vi "JSON FASES GEN.vi"(5 "time":u32, 7 "Tension":dbl, 8 "error in":errorcluster, 9 "Fase":u32, 10 "Corriente":dbl, 11 "Potencia":dbl) -> (0 "error out":errorcluster, 3 "JSON Object out":refnum<class "JSON Object.lvclass">)   [LabVIEW 2015]
uses:
  <vilib>/addons/JSON API/Get Polymorphic/JSON GetSet.lvlib
  <vilib>/addons/JSON API/JSON Scalar/Set SGL.vi
  <vilib>/addons/JSON API/JSON Scalar/JSON Scalar.lvclass
  <vilib>/addons/JSON API/JSON Object/Set Object Item by name.vi
  <vilib>/addons/JSON API/JSON Object/JSON Object.lvclass
  <vilib>/addons/JSON API/JSON Scalar/Set DBL.vi
  <vilib>/addons/JSON API/JSON Scalar/Set U32.vi
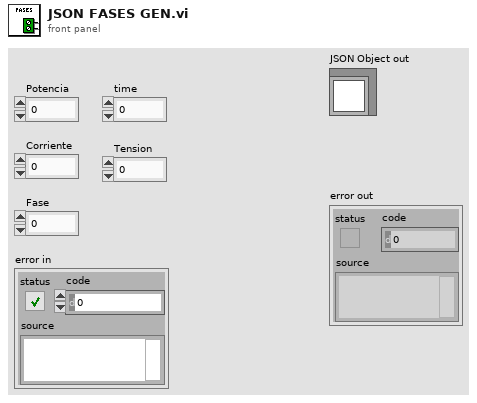
[diagram p1: front panel]
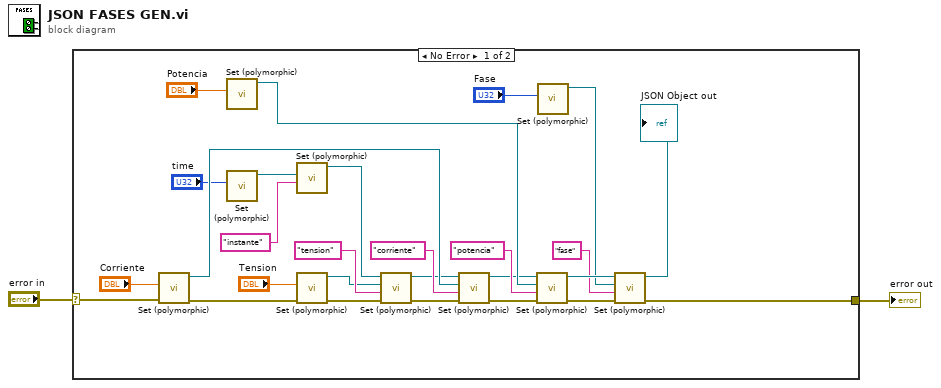
[diagram p0: block diagram]
diagram:
  n1 = case shown="No Error" "error in" {
    selector: "error in" -> [w3 w30]
    tunnel: [w11 w30] -> w2
    frame No Error {
      n2 = call-poly <vilib>:"Set (polymorphic).vi"("error in (no error)"=w3, "Numeric"="Corriente") -> ("error out"=w4:errorcluster, "JSON Scalar out"=w19:refnum<class "JSON Scalar.lvclass">)  [unwired: 8 in]
      n3 = call-poly <vilib>:"Set (polymorphic).vi"("Numeric"="Potencia") -> ("JSON Scalar out"=w22:refnum<class "JSON Scalar.lvclass">)  [unwired: 9 in, 1 out]
      n4 = call-poly <vilib>:"Set (polymorphic).vi"("Numeric"="time") -> ("JSON Scalar out"=w7:refnum<class "JSON Scalar.lvclass">)  [unwired: 9 in, 1 out]
      n5 = call-poly <vilib>:"Set (polymorphic).vi"("name"="instante", "Value"=w7) -> ("JSON Object out"=w5:refnum<class "JSON Object.lvclass">)  [unwired: 7 in, 2 out]
      n6 = call-poly <vilib>:"Set (polymorphic).vi"("error in (no error)"=w4, "Numeric"="Tension") -> ("error out"=w15:errorcluster, "JSON Scalar out"=w13:refnum<class "JSON Scalar.lvclass">)  [unwired: 8 in]
      n7 = call-poly <vilib>:"Set (polymorphic).vi"("error in (no error)"=w15, "name"="tension", "Value"=w13, "JSON Object in"=w5) -> ("error out"=w18:errorcluster, "JSON Object out"=w16:refnum<class "JSON Object.lvclass">)  [unwired: 5 in, 1 out]
      n8 = call-poly <vilib>:"Set (polymorphic).vi"("error in (no error)"=w18, "name"="corriente", "Value"=w19, "JSON Object in"=w16) -> ("error out"=w28:errorcluster, "JSON Object out"=w20:refnum<class "JSON Object.lvclass">)  [unwired: 5 in, 1 out]
      n9 = call-poly <vilib>:"Set (polymorphic).vi"("error in (no error)"=w28, "name"="potencia", "Value"=w22, "JSON Object in"=w20) -> ("error out"=w29:errorcluster, "JSON Object out"=w27:refnum<class "JSON Object.lvclass">)  [unwired: 5 in, 1 out]
      n10 = call-poly <vilib>:"Set (polymorphic).vi"("Numeric"="Fase") -> ("JSON Scalar out"=w26:refnum<class "JSON Scalar.lvclass">)  [unwired: 9 in, 1 out]
      n11 = call-poly <vilib>:"Set (polymorphic).vi"("error in (no error)"=w29, "name"="fase", "Value"=w26, "JSON Object in"=w27) -> ("error out"=w11:errorcluster, "JSON Object out"=→"JSON Object out":refnum<class "JSON Object.lvclass">)  [unwired: 5 in, 1 out]
    }
    frame Error {
    }
  }
  "error out" <- w2
